vi "Obtain Module Semaphore.vi"(8 "error in":errorcluster) -> (0 "error out":errorcluster, 1 "created new?":bool, 3 "semaphore":T1)   [LabVIEW 2026, in "Device Manager.lvlib"]
doc: "Obtain this module's Semaphore.\n_____\nBased on DQMH Dev Tools: Project Template 7.1.2.1547."
uses:
  Device Manager.lvlib
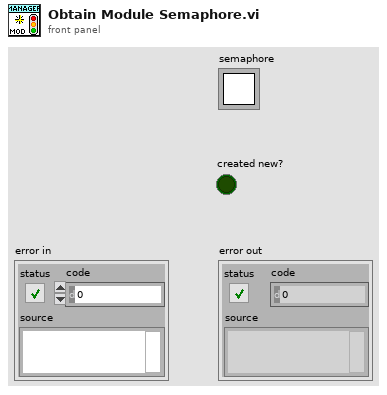
[diagram p1: front panel]
types:
  T1 = typedef "Semaphore RefNum" = refnum<k1>
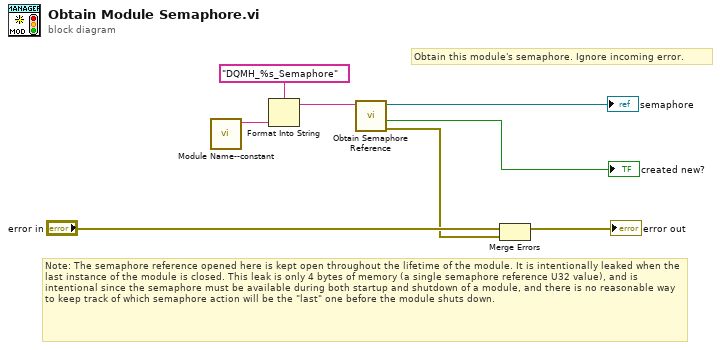
[diagram p0: block diagram]
diagram:
  # "Note: The semaphore reference opened here is kept open throughout the lifetime of the module. It is intentionally leaked when the last instance of the module is closed. This leak is only 4 bytes of memory (a single semaphore reference U32 value), and is intentional since the semaphore must be available during both startup and shutdown of a module, and there is no reasonable way to keep track of which semaphore action will be the \"last\" one before the module shuts down."
  # "Obtain this module's semaphore. Ignore incoming error."
  n1 = call "Module Name--constant.vi"() -> ("Module Name"=w4:string)  [unwired: 11 in]
  n2 = Format Into String(format string="DQMH_%s_Semaphore", w4) -> (resulting string=w3:string)  [unwired: 2 in, 1 out]
  n3 = call <vilib>:"Obtain Semaphore Reference.vi"("name (unnamed)"=w3) -> ("error out"=w7:errorcluster, "created new"=→"created new?":bool, "semaphore"=→"semaphore":T1)  [unwired: 4 in]
  n4 = Merge Errors("error in", w7) -> (→"error out":errorcluster)
